vi "Truncate full path to a given string length.vi"(5 "Max. Number of allowable characters":i32=60, 7 "Truncation Option":T1(ring), 11 "Full Path":path) -> (2 "Output String":string)   [LabVIEW 2022 SP3, in "Generic Utilities.lvclass"]
uses:
  Generic Utilities.lvclass
panel:
  out "length":i32
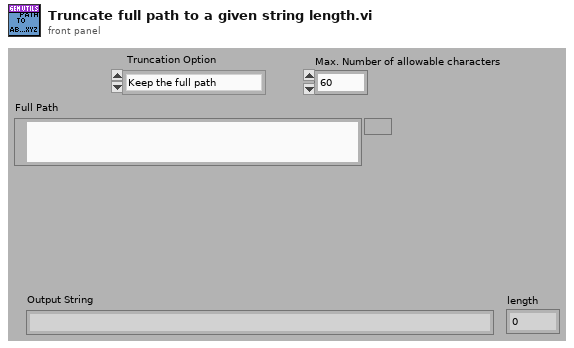
[diagram p1: front panel]
types:
  T1 = enum16{"Keep the full path", "File name ONLY", "Keep the full path - Force file name display"}
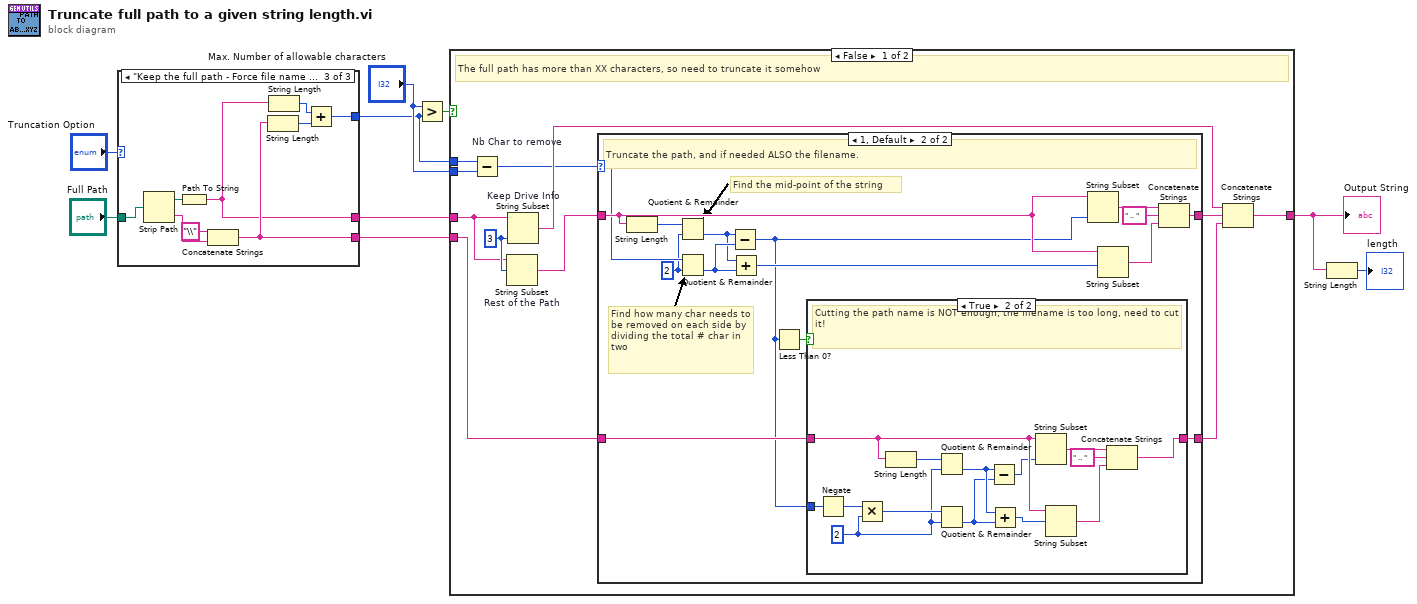
[diagram p0: block diagram]
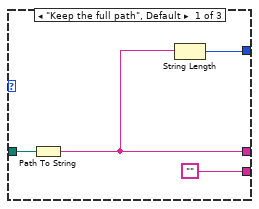
[diagram p2: hidden frame]
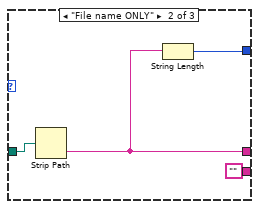
[diagram p3: hidden frame]
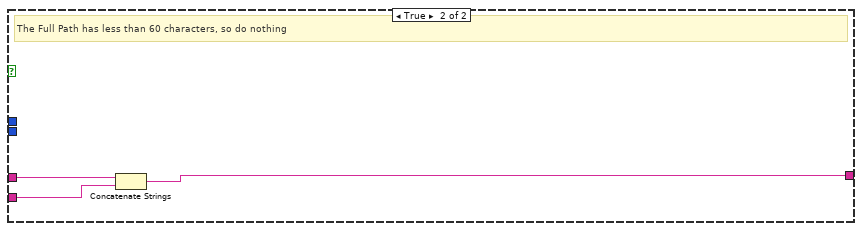
[diagram p6: hidden frame]
diagram:
  n1 = case shown="\"Keep the full path - Force file name display\"" "Truncation Option" {
    tunnel: "Full Path" -> [w13 w17 w20]
    tunnel: [w11 w15 w19] -> w6
    tunnel: ["" "" w22] -> w5
    tunnel: [w10 w14 w18] -> w1
    frame "Keep the full path", Default {
      n2 = Path To String(path=w13) -> (string=w11:string)
      n3 = String Length(string=w11) -> (length=w10:i32)
    }
    frame "File name ONLY" {
      n4 = Strip Path(path=w17) -> (name=w15:string)  [unwired: 1 out]
      n5 = String Length(string=w15) -> (length=w14:i32)
    }
    frame "Keep the full path - Force file name display" {
      n6 = Strip Path(path=w20) -> (stripped path=w26:path, name=w25:string)
      n7 = Path To String(path=w26) -> (string=w19:string)
      n8 = Concatenate Strings("\\", w25) -> (w22:string)
      n9 = String Length(string=w22) -> (length=w23:i32)
      n10 = String Length(string=w19) -> (length=w21:i32)
      n11 = Add(x=w21, y=w23) -> (x+y=w18:i32)
    }
  }
  n12 = Greater?(x="Max. Number of allowable characters", y=w1) -> (0:w9:bool)
  n13 = case shown="False" w9 {
    tunnel: [w36 w70] -> w4
    tunnel: w6 -> [w32 w72]
    tunnel: w5 -> [w29 w71]
    tunnel: "Max. Number of allowable characters" -> [w34 _]
    tunnel: w1 -> [w30 _]
    frame False {
      w33 = 3 ("length (rest)")
      # "The full path has more than XX characters, so need to truncate it somehow"
      n14 = Subtract "Nb Char to remove"(x=w30, y=w34) -> (x-y=w27:i32)
      n15 = String Subset "Rest of the Path"(string=w32, offset (0)=w33) -> (substring=w31:string)  [unwired: 1 in]
      n16 = String Subset "Keep Drive Info"(string=w32, length (rest)=w33) -> (substring=w35:string)  [unwired: 1 in]
      n17 = case shown="1, Default" w27 {
        selector: w27 -> [_ w43]
        tunnel: w31 -> [w39 w44]
        tunnel: [w39 w51] -> w37
        tunnel: [w38 w49] -> w28
        tunnel: w29 -> [w38 w48]
        frame 0 {
          # "Do NOT do nothing because the string is already shorter than the desired truncation"
        }
        frame 1, Default {
          w40 = 2 ("y")
          # "Find how many char needs to be removed on each side by dividing the total # char in two"
          # "Find the mid-point of the string"
          # "Truncate the path, and if needed ALSO the filename."
          n18 = String Length(string=w44) -> (length=w45:i32)
          n19 = Quotient & Remainder(x=w45, y=w40) -> (floor(x/y)=w46:i32)  [unwired: 1 out]
          n20 = Quotient & Remainder(x=w43, y=w40) -> (floor(x/y)=w47:i32)  [unwired: 1 out]
          n21 = Subtract(x=w46, y=w47) -> (x-y=w41:i32)
          n22 = Add(x=w46, y=w47) -> (x+y=w42:i32)
          n23 = Less Than 0?(x=w41) -> (x < 0?=w50:bool)
          n24 = case shown="True" w50 {
            tunnel: [w55 w58] -> w49
            tunnel: w48 -> [w55 w61]
            tunnel: w41 -> [_ w66]
            frame False {
            }
            frame True {
              w56 = 2 ("y")
              # "Cutting the path name is NOT enough, the filename is too long, need to cut it!"
              n25 = Negate(x=w66) -> (-x=w65:i32)
              n26 = Multiply(x=w65, y=w56) -> (x*y=w57:i32)
              n27 = String Length(string=w61) -> (length=w69:i32)
              n28 = Quotient & Remainder(x=w69, y=w56) -> (floor(x/y)=w68:i32)  [unwired: 1 out]
              n29 = Quotient & Remainder(x=w57, y=w56) -> (floor(x/y)=w67:i32)  [unwired: 1 out]
              n30 = Subtract(x=w68, y=w67) -> (x-y=w60:i32)
              n31 = Add(x=w68, y=w67) -> (x+y=w59:i32)
              n32 = String Subset(string=w61, length (rest)=w60) -> (substring=w62:string)  [unwired: 1 in]
              n33 = String Subset(string=w61, offset (0)=w59) -> (substring=w64:string)  [unwired: 1 in]
              n34 = Concatenate Strings(w62, " .. " ("string"), w64) -> (w58:string)
            }
          }
          n35 = String Subset(string=w44, length (rest)=w41) -> (substring=w54:string)  [unwired: 1 in]
          n36 = String Subset(string=w44, offset (0)=w42) -> (substring=w52:string)  [unwired: 1 in]
          n37 = Concatenate Strings(w54, " .. " ("string"), w52) -> (w51:string)
        }
      }
      n38 = Concatenate Strings(w35, w37, w28) -> (w36:string)
    }
    frame True {
      # "The Full Path has less than 60 characters, so do nothing"
      n39 = Concatenate Strings(w72, w71) -> (w70:string)
    }
  }
  "Output String" <- w4
  n40 = String Length(string=w4) -> (length=→"length":i32)
